vi "Initialize.vi"(8 "error in (no error)":errorcluster, 11 "File in":refnum<class "File.lvclass">) -> (0 "error out":errorcluster, 2 "File Path":path, 3 "File out":refnum<class "File.lvclass">)   [LabVIEW 2019, in "File.lvclass"]
uses:
  File.lvclass
  File.lvclass/File.ctl
  Read Include time.vi
  Read File format.vi
  Read Root Data Folder.vi
  Read Index digits.vi
  Read File Prefix.vi
  Write Data File  Path.vi
  Write Settings File Path.vi
  Write Index  File Path.vi
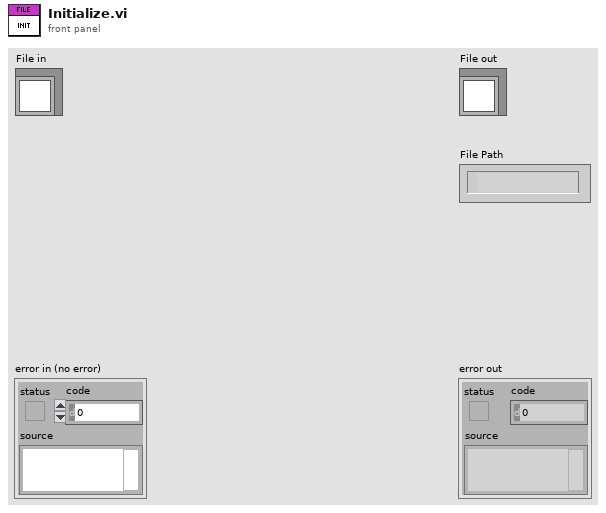
[diagram p1: front panel]
types:
  T1 = typedef "File formats.ctl" = enum16{"TDMS", "ASCII", "BINARY"}
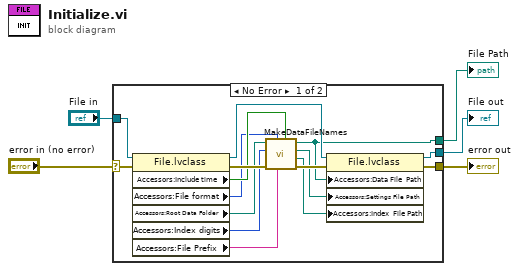
[diagram p0: block diagram]
diagram:
  n1 = case shown="No Error" "error in (no error)" {
    selector: "error in (no error)" -> [w20 w22]
    tunnel: [w13 w22] -> w2
    tunnel: [w12 w21] -> w3
    tunnel: "File in" -> [w17 w21]
    tunnel: [w11 _] -> w1
    frame No Error {
      n2 = property class="File.lvclass"(reference=w17, error in=w20) -> (reference out=w16:refnum<class "File.lvclass">, error out=w18:errorcluster, "Accessors:Include time"=w8:bool, "Accessors:File format"=w7:T1, "Accessors:Root Data Folder"=w14:path, "Accessors:Index digits"=w6:i32, "Accessors:File Prefix"=w15:string)
      n3 = call "MakeDataFileNames.vi"("Include time"=w8, "File Prefix"=w15, "File format"=w7, "Error In"=w18, "Index digits"=w6, "Root Data Folder"=w14) -> ("Error Out"=w19:errorcluster, "Index  File Path"=w9:path, "Settings File Path"=w10:path, "Data File  Path"=w11:path)  [unwired: 2 in]
      n4 = property class="File.lvclass"(reference=w16, error in=w19, "Accessors:Data File  Path"=w11, "Accessors:Settings File Path"=w10, "Accessors:Index  File Path"=w9) -> (reference out=w12:refnum<class "File.lvclass">, error out=w13:errorcluster)
    }
    frame Error {
    }
  }
  "error out" <- w2
  "File out" <- w3
  "File Path" <- w1
